vi "ReadButtonConfig.vi"(7 "section":string="AVN", 11 "数组 2":string[](array[string])=["ECALL", "FM/AM", "NAVI", "MENU", "BT", "VOL", "出仓", "播放", "上一首", "下一首", "EQ", "TUNE", "DVD", "SRC"]) -> (3 "数组":bool[](array[boolean]))   [LabVIEW 2013]
uses:
  GlobalValue.vi
  <vilib>/Utility/config.llb/Read Key (Boolean).vi
  <vilib>/Utility/config.llb/NI_LVConfig.lvlib
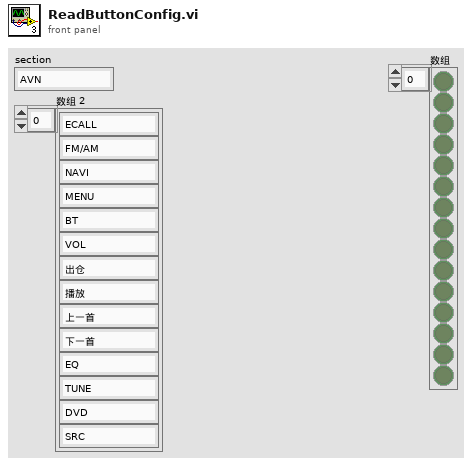
[diagram p1: front panel]
types:
  T1 = typedef "NI_LVConfig.lvlib/Config Data RefNum.ctl" = refnum<k1>
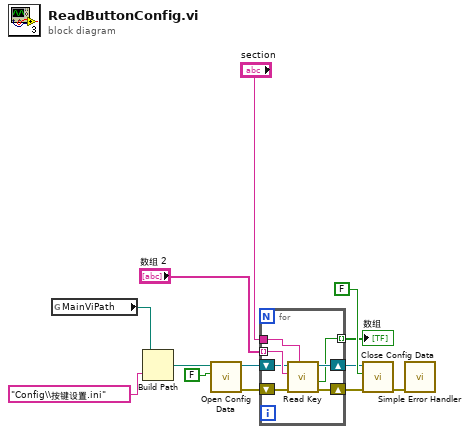
[diagram p0: block diagram]
diagram:
  n1 = global read "GlobalValue.vi" "MainViPath"() -> (w1:path)
  n2 = Build Path(base path=w1, name or relative path="Config\\按键设置.ini" ("名称或相对路径")) -> (appended path=w7:path)
  n3 = call <vilib>:"Open Config Data.vi"("create file if necessary (T)"=FALSE ("create file if necessary? (T)"), "configuration file path"=w7) -> ("error out"=w12:errorcluster, "refnum"=w11:T1)  [unwired: 7 in, 1 out]
  n4 = for {
    tunnel: "section" -> [w20]
    tunnel: "数组 2" -> [w19] mode=indexing
    shift-right: [w16] -> w6
    shift-left: w11 -> [w17]
    shift-right: [w15] -> w5
    shift-left: w12 -> [w18]
    tunnel: [w14] -> w2 mode=indexing
    n5 = call-poly <vilib>:"Read Key.vi"("section"=w20, "error in (no error)"=w18, "key"=w19, "refnum"=w17) -> ("error out"=w15:errorcluster, "value"=w14:bool, "refnum out"=w16:T1)  [unwired: 1 in, 4 out]
  }
  "数组" <- w2
  n6 = call <vilib>:"Close Config Data.vi"("error in (no error)"=w5, "write file if changed (T)"=FALSE ("write configuration file? (T)"), "refnum"=w6) -> ("error out"=w8:errorcluster)  [unwired: 8 out]
  n7 = call <vilib>:"Simple Error Handler.vi"("error in (no error)"=w8) -> ()  [unwired: 1 in, 8 out]
